vi "Get Int.vi"(8 "error in (no error)":errorcluster, 11 "IIntStatic in":refnum<class "IIntStatic (Global).lvclass">) -> (0 "error out":errorcluster, 2 "Int":i32, 3 "IIntStatic out":refnum<class "IIntStatic (Global).lvclass">)   [LabVIEW 2009, in "IIntStatic (Global).lvclass"]
uses:
  IIntStatic (Global).lvclass
  Numeric Test Object.lvclass
  Source/IUnknown Class/IUnknown.lvclass
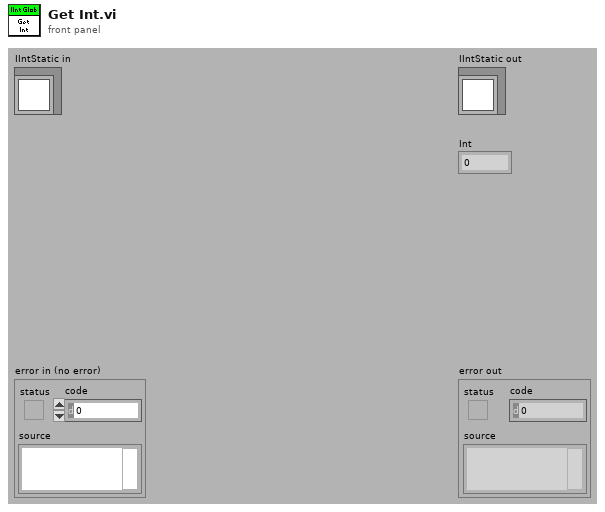
[diagram p1: front panel]
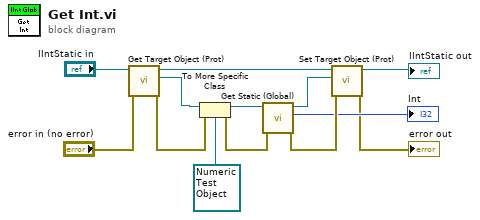
[diagram p0: block diagram]
diagram:
  n1 = call "Get Target Object (Prot).vi"("error in (no error)"="error in (no error)", "IUnknown in"="IIntStatic in") -> ("error out"=w12:errorcluster, "Target Object"=w13:refnum<class "Interfaceable.lvclass">, "IUnknown out"=w11:refnum<class "IIntStatic (Global).lvclass">)  [unwired: 7 in]
  n2 = To More Specific Class(target class=refnum<class "Numeric Test Object.lvclass"> refnum ("Numeric"), reference=w13, error in=w12) -> (specific class reference=w7:refnum<class "Numeric Test Object.lvclass">, error out=w6:errorcluster)
  n3 = call-dynamic "Get Static (Global).vi"("error in (no error)"=w6, "Numeric in"=w7) -> ("error out"=w5:errorcluster, "Int"=→"Int":i32, "Numeric out"=w4:refnum<class "Numeric Test Object.lvclass">)  [unwired: 7 in]
  n4 = call "Set Target Object (Prot).vi"("error in (no error)"=w5, "Target Object"=w4, "IUnknown in"=w11) -> ("error out"=→"error out":errorcluster, "IUnknown out"=→"IIntStatic out":refnum<class "IIntStatic (Global).lvclass">)  [unwired: 7 in]
